vi "Dashboard custom_bartender&global.vi"() -> ()   [LabVIEW 2017]
uses:
  C:/Users/IMR Lab/Documents/LabVIEW Data/UniversalRobotsSDK_LABView/LabVIEW/Examples/LabVIEW10/UnderAutomation.UniversalRobots.dll
  UnderAutomation.UniversalRobots.dll
  Global 1.vi
panel:
  out "3rd Order":bool
  out "2nd Order":bool
  out "1st Order":bool
  in  "stop":bool
  in  "TCP switch (server)":bool
  out "Rx":dbl
  out "Rz":dbl
  out "Ry":dbl
  out "Enabled":bool
  out "Port":i32
  in  "Move to particular posture":bool
  in  "Move to Zero position":bool
  out "Connected":bool
  in  "Robot IP(192.168.112.182)":string
  out "Connect error":errorcluster
  in  "Power on\nRelease brake":bool
  in  "Power off":bool
  in  "Connect":bool
  in  "Send script":bool
  in  "Script to execute":string
  out "Powered on":bool
  out "X":dbl
  out "Y":dbl
  out "Z":dbl
  out "License state":string
  # "movel(p[-0.0753945, -0.304532, 0.314608, -0.194623, 2.71667, -1.00228], a= 0.5, v=0.25)"
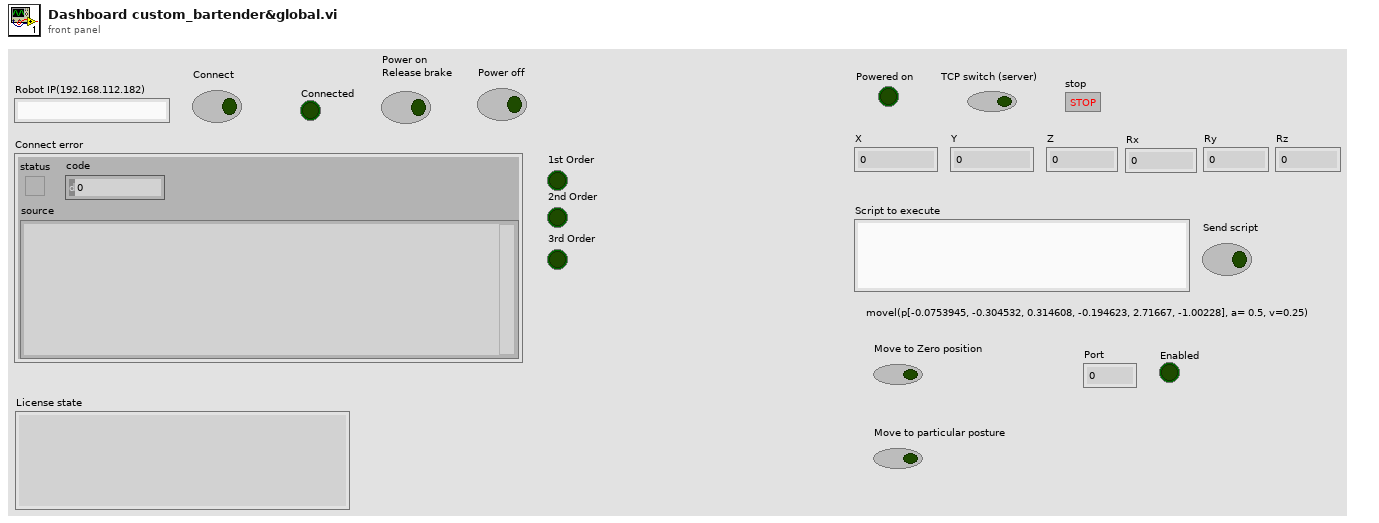
[diagram p1: front panel]
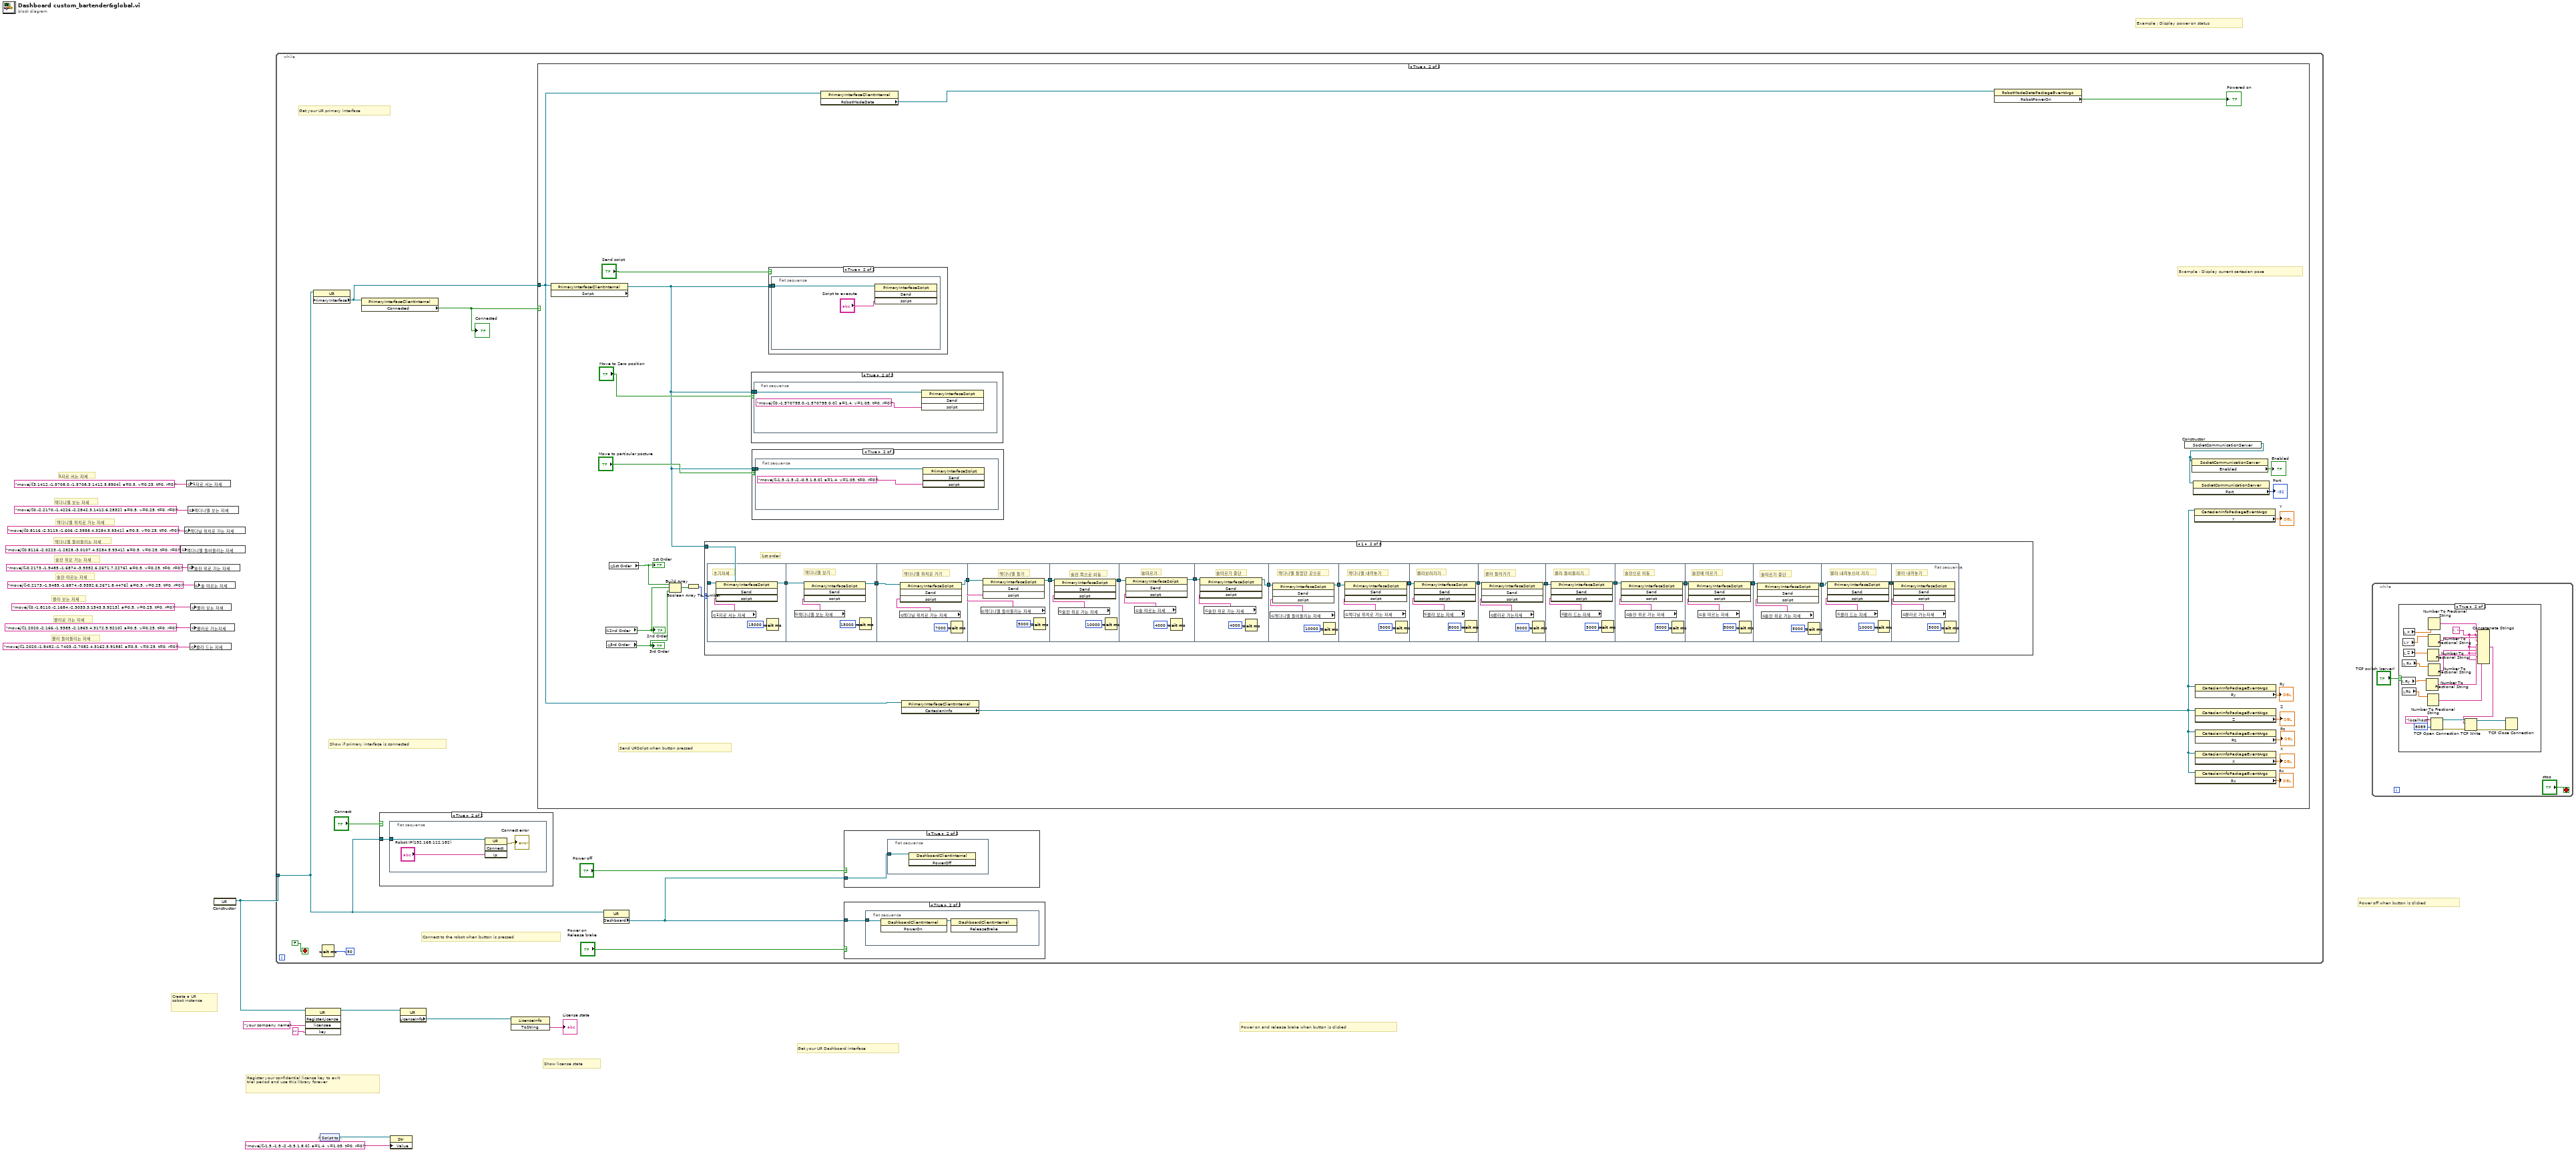
[diagram p0: block diagram]
diagram:
  # "콜라 들어올리는 자세"
  # "콜라로 가는 자세"
  # "콜라 보는 자세"
  # "술잔 따르는 자세"
  # "술잔 위로 가는 자세"
  # "잭다니엘 들어올리는 자세"
  # "잭다니엘 위치로 가는 자세"
  # "잭다니엘 보는 자세"
  # "1자로 서는 자세"
  # "Example : Display power on status"
  # "Create a UR\ncobot instance"
  # "Show license state"
  # "Register your confidential license key to exit\ntrial period and use this library forever"
  # "Power off when button is clicked"
  # "Power on and release brake when button is clicked"
  # "Get your UR Dashboard interface"
  n1 = global write "Global 1.vi" "잭다니엘 들어올리는 자세"("movej([0.8116,-2.0223,-1.2828,-3.0107,4.3284,5.9341], a=0.5, v=0.25, t=0, r=0)") -> ()
  n2 = global write "Global 1.vi" "잭다닐 위치로 가는 자세"("movej([0.8116,-2.3119,-1.606,-2.3958,4.3284,5.9341], a=0.5, v=0.25, t=0, r=0)") -> ()
  n3 = global write "Global 1.vi" "1자로 서는 자세"("movej([3.1412,-1.5708,0,-1.5708,3.1412,5.8904], a=0.5, v=0.25, t=0, r=0)") -> ()
  n4 = global write "Global 1.vi" "술잔 위로 가는 자세"("movej([-0.2173,-1.9485,-1.6874,-3.9352,6.2671,7.2276], a=0.5, v=0.25, t=0, r=0)") -> ()
  n5 = global write "Global 1.vi" "잭다니엘 보는 자세"("movej([0,-2.2170,-1.4226,-2.2842,3.1412,6.2832], a=0.5, v=0.25, t=0, r=0)") -> ()
  n6 = global write "Global 1.vi" "콜라 드는 자세"("movej([1.2020,-1.8452,-1.7403,-2.7082,4.3162,5.9158], a=0.5, v=0.25, t=0, r=0)") -> ()
  n7 = global write "Global 1.vi" "콜라 보는 자세"("movej([0,-1.8110,-2.1684,-2.3033,3.1543,5.9213], a=0.5, v=0.25, t=0, r=0)") -> ()
  n8 = global write "Global 1.vi" "콜라로 가는자세"("movej([1.2020,-2.166,-1.9385,-2.1863,4.3172,5.9210], a=0.5, v=0.25, t=0, r=0)") -> ()
  n9 = global write "Global 1.vi" "술 따르는 자세"("movej([-0.2173,-1.9485,-1.6874,-3.9352,6.2671,8.4476], a=0.5, v=0.25, t=0, r=0)") -> ()
  n10 = constructor class="UR"() -> (reference out=w12:refnum<k24>)  [unwired: 3 in, 2 out]
  n11 = while {
    tunnel: w12 -> [w18]
    stop <- FALSE stop-if-true
    # "Connect to the robot when button is pressed"
    # "Show if primary interface is connected"
    # "Get your UR primary interface"
    n12 = property class="UR"(reference=w18) -> ("PrimaryInterface"=w21:refnum<k24>)  [unwired: 1 in, 2 out]
    n13 = Wait (ms)(milliseconds to wait=u32 50) -> ()  [unwired: 1 out]
    n14 = property class="PrimaryInterfaceClientInternal"(reference=w21) -> ("Connected"=w20:bool)  [unwired: 1 in, 2 out]
    "Connected" <- w20
    n15 = case shown="True" "Connect" {
      tunnel: w18 -> [_ w147]
      frame False {
      }
      frame True {
        n16 = flat-sequence {
          tunnel: w147 -> [w149]
          frame #0 {
            n17 = invoke class="UR" method="Connect"(reference=w149, "ip"="Robot IP(192.168.112.182)") -> (error out=→"Connect error":errorcluster)  [unwired: 2 in, 3 out]
          }
        }
      }
    }
    n18 = case shown="True" w20 {
      tunnel: w21 -> [_ w42]
      frame False {
      }
      frame True {
        # "Send URScript when button pressed"
        # "Example : Display current cartesian pose"
        n19 = property class="PrimaryInterfaceClientInternal"(reference=w42) -> ("Script"=w27:refnum<k24>)  [unwired: 1 in, 2 out]
        n20 = global read "Global 1.vi" "2nd Order"() -> (w30:bool)
        "2nd Order" <- w30
        n21 = global read "Global 1.vi" "3rd Order"() -> (w29:bool)
        "3rd Order" <- w29
        n22 = global read "Global 1.vi" "1st Order"() -> (w31:bool)
        "1st Order" <- w31
        n23 = Build Array(w31, w30, w29) -> (w32:bool[])
        n24 = Boolean Array To Number(Boolean array=w32) -> (number=w28:u32)
        n25 = case shown="1" w28 {
          tunnel: w27 -> [_ w65 _ _ _ _ _ _]
          frame 0, Default {
          }
          frame 1 {
            # "1st order"
            n26 = flat-sequence {
              tunnel: w65 -> [w69]
              tunnel: [w68] -> w64
              tunnel: w64 -> [w73]
              tunnel: [w71] -> w50
              tunnel: w50 -> [w77]
              tunnel: [w74] -> w49
              tunnel: w49 -> [w79]
              tunnel: [w78] -> w63
              tunnel: w63 -> [w83]
              tunnel: [w82] -> w62
              tunnel: w62 -> [w88]
              tunnel: [w86] -> w61
              tunnel: w61 -> [w91]
              tunnel: [w90] -> w60
              tunnel: w60 -> [w96]
              tunnel: [w94] -> w59
              tunnel: w59 -> [w99]
              tunnel: [w98] -> w58
              tunnel: w58 -> [w103]
              tunnel: [w102] -> w57
              tunnel: w57 -> [w107]
              tunnel: [w106] -> w56
              tunnel: w56 -> [w111]
              tunnel: [w110] -> w55
              tunnel: w55 -> [w115]
              tunnel: [w114] -> w54
              tunnel: w54 -> [w119]
              tunnel: [w118] -> w53
              tunnel: w53 -> [w123]
              tunnel: [w122] -> w52
              tunnel: w52 -> [w127]
              tunnel: [w126] -> w51
              tunnel: w51 -> [w130]
              frame #0 {
                # "초기자세"
                n27 = global read "Global 1.vi" "1자로 서는 자세"() -> (w67:string)
                n28 = invoke class="PrimaryInterfaceScript" method="Send"(reference=w69, "script"=w67) -> (reference out=w68:refnum<k24>)  [unwired: 2 in, 3 out]
                n29 = Wait (ms)(milliseconds to wait=u32 15000) -> ()  [unwired: 1 out]
              }
              frame #1 {
                # "잭다니엘 보기"
                n30 = global read "Global 1.vi" "잭다니엘 보는 자세"() -> (w72:string)
                n31 = invoke class="PrimaryInterfaceScript" method="Send"(reference=w73, "script"=w72) -> (reference out=w71:refnum<k24>)  [unwired: 2 in, 3 out]
                n32 = Wait (ms)(milliseconds to wait=u32 15000) -> ()  [unwired: 1 out]
              }
              frame #2 {
                # "잭다니엘 위치로 가기"
                n33 = global read "Global 1.vi" "잭다닐 위치로 가는 자세"() -> (w76:string)
                n34 = invoke class="PrimaryInterfaceScript" method="Send"(reference=w77, "script"=w76) -> (reference out=w74:refnum<k24>)  [unwired: 2 in, 3 out]
                n35 = Wait (ms)(milliseconds to wait=u32 7000) -> ()  [unwired: 1 out]
              }
              frame #3 {
                # "잭다니엘 들기"
                n36 = global read "Global 1.vi" "잭다니엘 들어올리는 자세"() -> (w81:string)
                n37 = invoke class="PrimaryInterfaceScript" method="Send"(reference=w79, "script"=w81) -> (reference out=w78:refnum<k24>)  [unwired: 2 in, 3 out]
                n38 = Wait (ms)(milliseconds to wait=u32 5000) -> ()  [unwired: 1 out]
              }
              frame #4 {
                # "술잔 쪽으로 이동"
                n39 = global read "Global 1.vi" "술잔 위로 가는 자세"() -> (w84:string)
                n40 = invoke class="PrimaryInterfaceScript" method="Send"(reference=w83, "script"=w84) -> (reference out=w82:refnum<k24>)  [unwired: 2 in, 3 out]
                n41 = Wait (ms)(milliseconds to wait=u32 10000) -> ()  [unwired: 1 out]
              }
              frame #5 {
                # "술따르기"
                n42 = global read "Global 1.vi" "술 따르는 자세"() -> (w87:string)
                n43 = invoke class="PrimaryInterfaceScript" method="Send"(reference=w88, "script"=w87) -> (reference out=w86:refnum<k24>)  [unwired: 2 in, 3 out]
                n44 = Wait (ms)(milliseconds to wait=u32 4000) -> ()  [unwired: 1 out]
              }
              frame #6 {
                # "술따르기 중단"
                n45 = global read "Global 1.vi" "술잔 위로 가는 자세"() -> (w92:string)
                n46 = invoke class="PrimaryInterfaceScript" method="Send"(reference=w91, "script"=w92) -> (reference out=w90:refnum<k24>)  [unwired: 2 in, 3 out]
                n47 = Wait (ms)(milliseconds to wait=u32 4000) -> ()  [unwired: 1 out]
              }
              frame #7 {
                # "잭다니엘 들었던 곳으로"
                n48 = global read "Global 1.vi" "잭다니엘 들어올리는 자세"() -> (w95:string)
                n49 = invoke class="PrimaryInterfaceScript" method="Send"(reference=w96, "script"=w95) -> (reference out=w94:refnum<k24>)  [unwired: 2 in, 3 out]
                n50 = Wait (ms)(milliseconds to wait=u32 10000) -> ()  [unwired: 1 out]
              }
              frame #8 {
                # "잭다니엘 내려놓기"
                n51 = global read "Global 1.vi" "잭다닐 위치로 가는 자세"() -> (w101:string)
                n52 = invoke class="PrimaryInterfaceScript" method="Send"(reference=w99, "script"=w101) -> (reference out=w98:refnum<k24>)  [unwired: 2 in, 3 out]
                n53 = Wait (ms)(milliseconds to wait=u32 5000) -> ()  [unwired: 1 out]
              }
              frame #9 {
                # "콜라보러가기"
                n54 = global read "Global 1.vi" "콜라 보는 자세"() -> (w105:string)
                n55 = invoke class="PrimaryInterfaceScript" method="Send"(reference=w103, "script"=w105) -> (reference out=w102:refnum<k24>)  [unwired: 2 in, 3 out]
                n56 = Wait (ms)(milliseconds to wait=u32 8000) -> ()  [unwired: 1 out]
              }
              frame #10 {
                # "콜라 들러가기"
                n57 = global read "Global 1.vi" "콜라로 가는자세"() -> (w109:string)
                n58 = invoke class="PrimaryInterfaceScript" method="Send"(reference=w107, "script"=w109) -> (reference out=w106:refnum<k24>)  [unwired: 2 in, 3 out]
                n59 = Wait (ms)(milliseconds to wait=u32 8000) -> ()  [unwired: 1 out]
              }
              frame #11 {
                # "콜라 들어올리기"
                n60 = global read "Global 1.vi" "콜라 드는 자세"() -> (w113:string)
                n61 = invoke class="PrimaryInterfaceScript" method="Send"(reference=w111, "script"=w113) -> (reference out=w110:refnum<k24>)  [unwired: 2 in, 3 out]
                n62 = Wait (ms)(milliseconds to wait=u32 5000) -> ()  [unwired: 1 out]
              }
              frame #12 {
                # "술잔으로 이동"
                n63 = global read "Global 1.vi" "술잔 위로 가는 자세"() -> (w117:string)
                n64 = invoke class="PrimaryInterfaceScript" method="Send"(reference=w115, "script"=w117) -> (reference out=w114:refnum<k24>)  [unwired: 2 in, 3 out]
                n65 = Wait (ms)(milliseconds to wait=u32 8000) -> ()  [unwired: 1 out]
              }
              frame #13 {
                # "술잔에 따르기"
                n66 = global read "Global 1.vi" "술 따르는 자세"() -> (w121:string)
                n67 = invoke class="PrimaryInterfaceScript" method="Send"(reference=w119, "script"=w121) -> (reference out=w118:refnum<k24>)  [unwired: 2 in, 3 out]
                n68 = Wait (ms)(milliseconds to wait=u32 5000) -> ()  [unwired: 1 out]
              }
              frame #14 {
                # "술따르기 중단"
                n69 = global read "Global 1.vi" "술잔 위로 가는 자세"() -> (w125:string)
                n70 = invoke class="PrimaryInterfaceScript" method="Send"(reference=w123, "script"=w125) -> (reference out=w122:refnum<k24>)  [unwired: 2 in, 3 out]
                n71 = Wait (ms)(milliseconds to wait=u32 5000) -> ()  [unwired: 1 out]
              }
              frame #15 {
                # "콜라 내려놓으러 가기"
                n72 = global read "Global 1.vi" "콜라 드는 자세"() -> (w129:string)
                n73 = invoke class="PrimaryInterfaceScript" method="Send"(reference=w127, "script"=w129) -> (reference out=w126:refnum<k24>)  [unwired: 2 in, 3 out]
                n74 = Wait (ms)(milliseconds to wait=u32 10000) -> ()  [unwired: 1 out]
              }
              frame #16 {
                # "콜라 내려놓기"
                n75 = global read "Global 1.vi" "콜라로 가는자세"() -> (w132:string)
                n76 = invoke class="PrimaryInterfaceScript" method="Send"(reference=w130, "script"=w132) -> ()  [unwired: 2 in, 4 out]
                n77 = Wait (ms)(milliseconds to wait=u32 5000) -> ()  [unwired: 1 out]
              }
            }
          }
          frame 2 {
            # "2nd order"
          }
          frame 3 {
            # "multi order"
          }
          frame 4 {
            # "3rd order"
          }
          frame 5 {
            # "multi order"
          }
          frame 6 {
            # "multi order"
          }
          frame 7 {
            # "multi order"
          }
        }
        n78 = case shown="True" "Move to Zero position" {
          tunnel: w27 -> [_ w136]
          frame False {
          }
          frame True {
            n79 = flat-sequence {
              tunnel: w136 -> [w138]
              frame #0 {
                n80 = invoke class="PrimaryInterfaceScript" method="Send"(reference=w138, "script"="movej([0,-1.570795,0,-1.570795,0,0], a=1.4, v=1.05, t=0, r=0)") -> ()  [unwired: 2 in, 4 out]
              }
            }
          }
        }
        n81 = case shown="True" "Move to particular posture" {
          tunnel: w27 -> [_ w133]
          frame False {
          }
          frame True {
            n82 = flat-sequence {
              tunnel: w133 -> [w135]
              frame #0 {
                n83 = invoke class="PrimaryInterfaceScript" method="Send"(reference=w135, "script"="movej([-1.5,-1.5,-2,-0.5,1.8,0], a=1.4, v=1.05, t=0, r=0)") -> ()  [unwired: 2 in, 4 out]
              }
            }
          }
        }
        n84 = case shown="True" "Send script" {
          tunnel: w27 -> [_ w139]
          frame False {
          }
          frame True {
            n85 = flat-sequence {
              tunnel: w139 -> [w141]
              frame #0 {
                n86 = invoke class="PrimaryInterfaceScript" method="Send"(reference=w141, "script"="Script to execute") -> ()  [unwired: 2 in, 4 out]
              }
            }
          }
        }
        n87 = property class="PrimaryInterfaceClientInternal"(reference=w42) -> ("RobotModeData"=w47:refnum<k24>)  [unwired: 1 in, 2 out]
        n88 = property class="PrimaryInterfaceClientInternal"(reference=w42) -> ("CartesianInfo"=w34:refnum<k24>)  [unwired: 1 in, 2 out]
        n89 = property class="RobotModeDataPackageEventArgs"(reference=w47) -> ("RobotPowerOn"=→"Powered on":bool)  [unwired: 1 in, 2 out]
        n90 = constructor class="SocketCommunicationServer"() -> (reference out=w39:refnum<k24>)  [unwired: 3 in, 2 out]
        n91 = property class="SocketCommunicationServer"(reference=w39) -> ("Enabled"=→"Enabled":bool)  [unwired: 1 in, 2 out]
        n92 = property class="SocketCommunicationServer"(reference=w39) -> ("Port"=→"Port":i32)  [unwired: 1 in, 2 out]
        n93 = property class="CartesianInfoPackageEventArgs"(reference=w34) -> ("Y"=→"Y":dbl)  [unwired: 1 in, 2 out]
        n94 = property class="CartesianInfoPackageEventArgs"(reference=w34) -> ("Ry"=→"Ry":dbl)  [unwired: 1 in, 2 out]
        n95 = property class="CartesianInfoPackageEventArgs"(reference=w34) -> ("Z"=→"Z":dbl)  [unwired: 1 in, 2 out]
        n96 = property class="CartesianInfoPackageEventArgs"(reference=w34) -> ("Rz"=→"Rz":dbl)  [unwired: 1 in, 2 out]
        n97 = property class="CartesianInfoPackageEventArgs"(reference=w34) -> ("X"=→"X":dbl)  [unwired: 1 in, 2 out]
        n98 = property class="CartesianInfoPackageEventArgs"(reference=w34) -> ("Rx"=→"Rx":dbl)  [unwired: 1 in, 2 out]
      }
    }
    n99 = property class="UR"(reference=w18) -> ("Dashboard"=w22:refnum<k24>)  [unwired: 1 in, 2 out]
    n100 = case shown="True" "Power off" {
      tunnel: w22 -> [_ w142]
      frame False {
      }
      frame True {
        n101 = flat-sequence {
          tunnel: w142 -> [w143]
          frame #0 {
            n102 = invoke class="DashboardClientInternal" method="PowerOff"(reference=w143) -> ()  [unwired: 2 in, 3 out]
          }
        }
      }
    }
    n103 = case shown="True" "Power on\nRelease brake" {
      tunnel: w22 -> [_ w144]
      frame False {
      }
      frame True {
        n104 = flat-sequence {
          tunnel: w144 -> [w146]
          frame #0 {
            n105 = invoke class="DashboardClientInternal" method="PowerOn"(reference=w146) -> (reference out=w145:refnum<k24>)  [unwired: 2 in, 2 out]
            n106 = invoke class="DashboardClientInternal" method="ReleaseBrake"(reference=w145) -> ()  [unwired: 2 in, 3 out]
          }
        }
      }
    }
  }
  n107 = invoke class="UR" method="RegisterLicense"(reference=w12, "licensee"="your company name", "key"="") -> (reference out=w14:refnum<k24>)  [unwired: 2 in, 4 out]
  n108 = control-ref of="Script to execute"() -> (w11:refnum<vi>)
  n109 = property class="Str"(reference=w11, "Value"="movej([-1.5,-1.5,-2,-0.5,1.8,0], a=1.4, v=1.05, t=0, r=0)") -> ()  [unwired: 1 in, 2 out]
  n110 = property class="UR"(reference=w14) -> ("LicenseInfo"=w13:refnum<k24>)  [unwired: 1 in, 2 out]
  n111 = invoke class="LicenseInfo" method="ToString"(reference=w13) -> ("ToString"=→"License state":string)  [unwired: 2 in, 2 out]
  n112 = while {
    stop <- "stop" stop-if-true
    n113 = case shown="True" "TCP switch (server)" {
      frame False {
      }
      frame True {
        w155 = ", "
        n114 = local read "Ry"() -> (w162:dbl)
        n115 = local read "Rz"() -> (w161:dbl)
        n116 = local read "Rx"() -> (w163:dbl)
        n117 = local read "Y"() -> (w165:dbl)
        n118 = local read "X"() -> (w166:dbl)
        n119 = local read "Z"() -> (w164:dbl)
        n120 = Number To Fractional String(number=w162) -> (F-format string=w156:string)  [unwired: 3 in]
        n121 = Number To Fractional String(number=w164) -> (F-format string=w158:string)  [unwired: 3 in]
        n122 = Number To Fractional String(number=w161) -> (F-format string=w154:string)  [unwired: 3 in]
        n123 = Number To Fractional String(number=w166) -> (F-format string=w160:string)  [unwired: 3 in]
        n124 = Number To Fractional String(number=w165) -> (F-format string=w159:string)  [unwired: 3 in]
        n125 = Number To Fractional String(number=w163) -> (F-format string=w157:string)  [unwired: 3 in]
        n126 = TCP Open Connection(address="localhost", remote port or service name=u16 8089) -> (connection ID=w170:refnum<k5>, error out=w169:errorcluster)  [unwired: 3 in]
        n127 = Concatenate Strings(w160, w155, w159, w155, w158, w155, w157, w155, w156, w155, w154) -> (w153:string)
        n128 = TCP Write(connection ID=w170, data in=w153, error in (no error)=w169) -> (connection ID out=w168:refnum<k5>, error out=w167:errorcluster)  [unwired: 1 in, 1 out]
        n129 = TCP Close Connection(connection ID=w168, error in (no error)=w167) -> ()  [unwired: 1 in, 2 out]
      }
    }
  }
